vi "Configure Baud Rate.vi"(8 "error in (no error)":errorcluster, 10 "baud rate":u32(ring)=9600 items=["9600"=9600, "19200"=19200, "38400"=38400], 11 "RRG in":refnum<class "PL Eltochpribor RRG.lvclass">) -> (0 "error out":errorcluster, 3 "RRG out":refnum<class "PL Eltochpribor RRG.lvclass">)   [LabVIEW 2015, in "PL Eltochpribor RRG.lvclass"]
doc: "Configures device communication baud rate."
uses:
  PL Eltochpribor RRG.lvclass
  <vilib>/plasmapper/PL Modbus Client/PL Modbus Client.lvclass
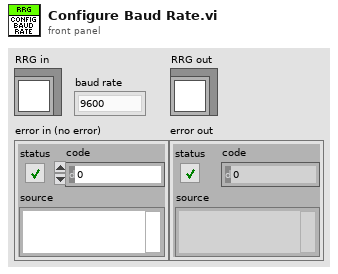
[diagram p1: front panel]
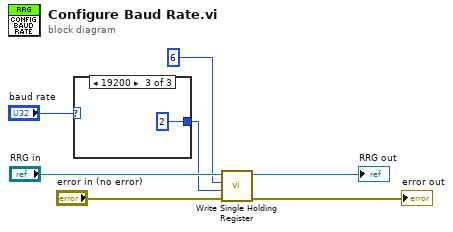
[diagram p0: block diagram]
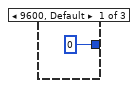
[diagram p2: hidden frame]
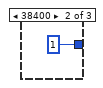
[diagram p3: hidden frame]
diagram:
  n1 = case shown="19200" "baud rate" {
    tunnel: [u16 0 ("value") u16 1 ("value") u16 2 ("value")] -> w1
    frame 9600, Default {
    }
    frame 38400 {
    }
    frame 19200 {
    }
  }
  n2 = call <vilib>:"Write Single Holding Register.vi"("error in (no error)"="error in (no error)", "value"=w1, "address"=u16 6, "MODBUS in"="RRG in") -> ("error out"=→"error out":errorcluster, "MODBUS out"=→"RRG out":refnum<class "PL Eltochpribor RRG.lvclass">)  [unwired: 6 in]
